vi "GetData.vi"(8 "error in (no error)":errorcluster, 11 "USB-9215 in":refnum<class "USB-9215.lvclass">) -> (0 "error out":errorcluster, 2 "Waveform":waveform(dbl), 3 "USB-9215 out":refnum<class "USB-9215.lvclass">)   [LabVIEW 2013, in "USB-9215.lvclass"]
uses:
  USB-9215.lvclass
  DAQSuper/DAQSuper.lvclass
  <vilib>/measure/NI_MABase.lvlib
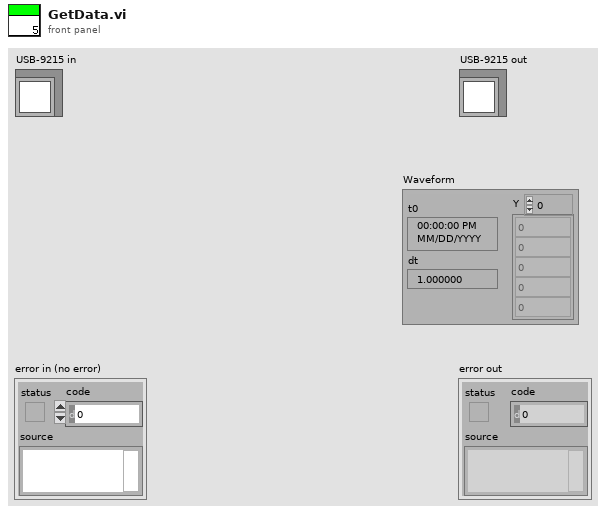
[diagram p1: front panel]
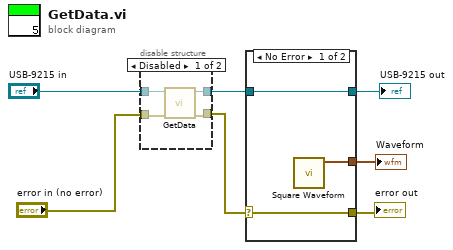
[diagram p0: block diagram]
diagram:
  n1 = disable-structure shown="Disabled" {
    disable-tunnel: "error in (no error)" -> [w11 w12]
    disable-tunnel: "USB-9215 in" -> [w10 w13]
    disable-tunnel: [w9 w12] -> w5
    disable-tunnel: [w8 w13] -> w2
    frame Disabled {
      n2 = call-parent "GetData.vi"("error in (no error)"=w11, "DAQSuper in"=w10) -> ("error out"=w9:errorcluster, "DAQSuper out"=w8:refnum<class "USB-9215.lvclass">)  [unwired: 7 in, 1 out]
    }
    frame Enabled {
    }
  }
  n3 = case shown="No Error" w5 {
    selector: w5 -> [w16 w17]
    tunnel: [w16 w17] -> w4
    tunnel: [w15 w18] -> w3
    tunnel: w2 -> [w15 w18]
    tunnel: [w14 _] -> w1
    frame No Error {
      n4 = call <vilib>:"Square Waveform.vi"() -> ("signal out"=w14:waveform(dbl))  [unwired: 10 in, 1 out]
    }
    frame Error {
    }
  }
  "error out" <- w4
  "USB-9215 out" <- w3
  "Waveform" <- w1
